vi "WhileLoop to Code.vi"(8 "error in":errorcluster, 10 "C code in":string, 11 "WhileLoop ref":refnum<vi>) -> (0 "error out":errorcluster, 2 "C code":string, 3 "terminals info":T1)   [LabVIEW 2014]
uses:
  <vilib>/regexp/Match Regular Expression.xnode
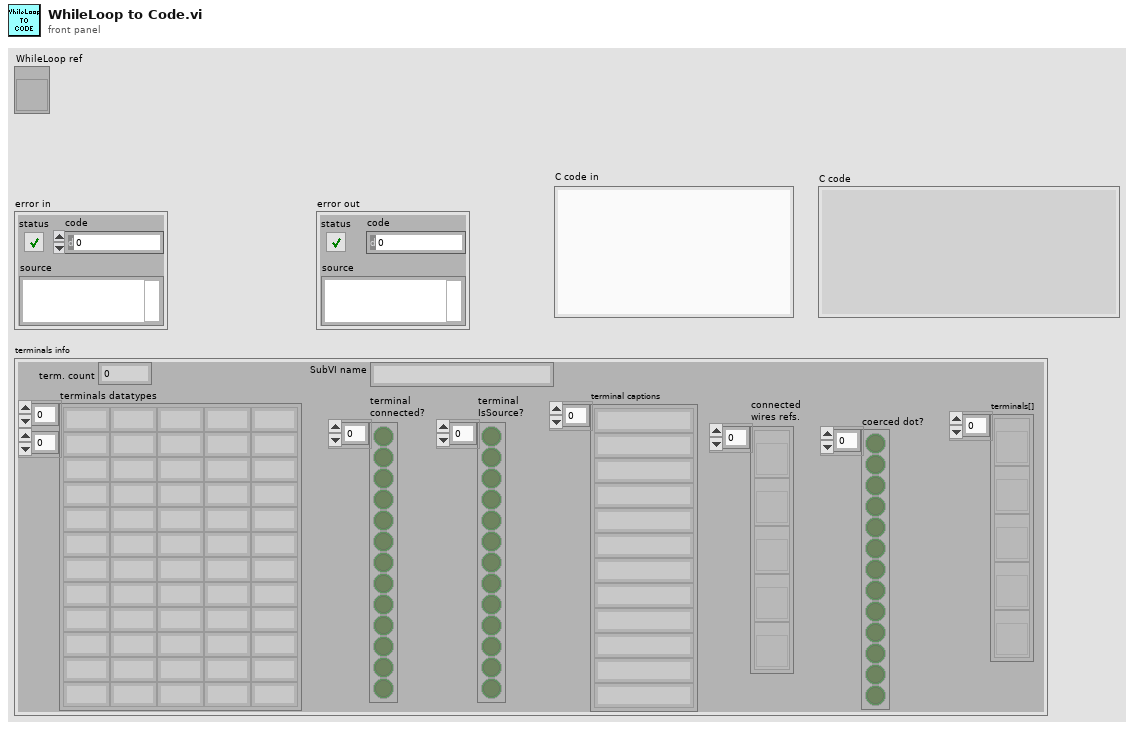
[diagram p1: front panel]
types:
  T1 = cluster{"terminals datatypes":string[][], "terminal\nconnected?":bool[], "terminal captions":string[], "term. count":i32, "terminal\nIsSource?":bool[], "SubVI name":string, "connected\nwires refs.":refnum<vi>[], "coerced dot?":bool[], "terminals[]":refnum<vi>[]}
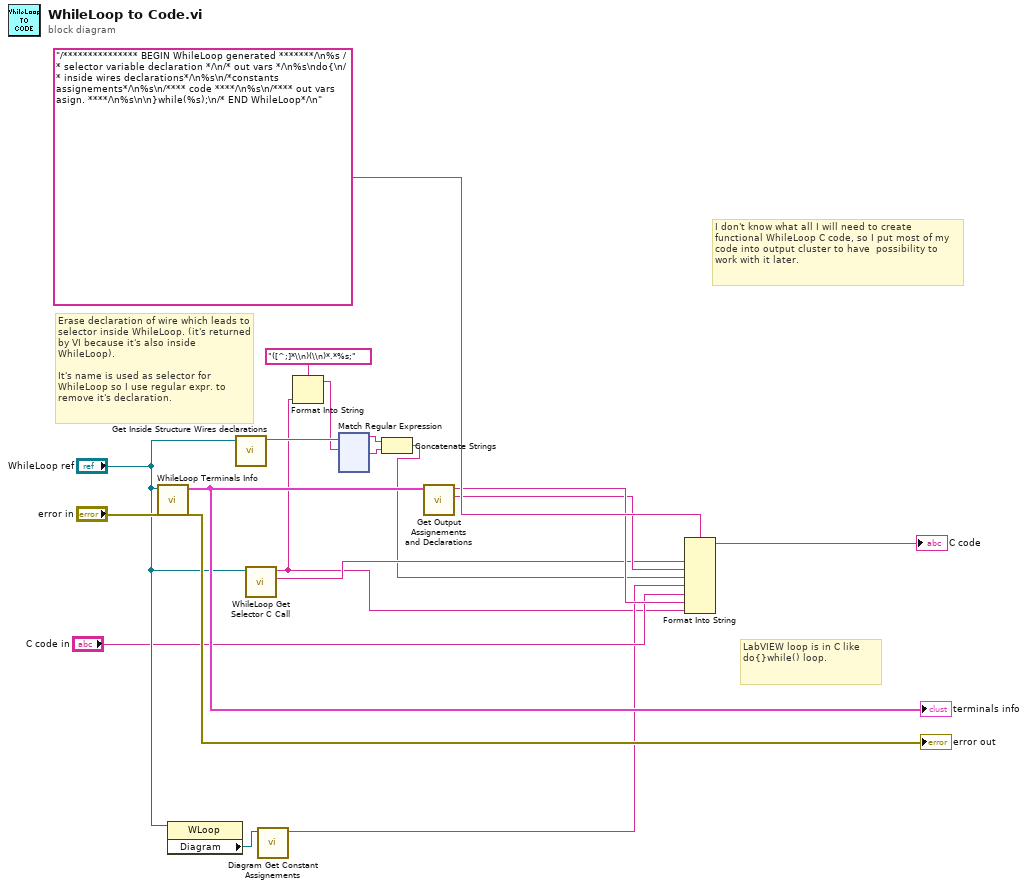
[diagram p0: block diagram]
diagram:
  # "Erase declaration of wire which leads to selector inside WhileLoop. (it's returned by VI because it's also inside WhileLoop).\n\nIt's name is used as selector for WhileLoop so I use regular expr. to remove it's declaration."
  # "I don't know what all I will need to create functional WhileLoop C code, so I put most of my code into output cluster to have  possibility to work with it later."
  # "LabVIEW loop is in C like do{}while() loop."
  n1 = call "WhileLoop Terminals Info.vi"("error in"="error in", "reference"="WhileLoop ref") -> ("error out"=→"error out":errorcluster, "output cluster"=w16:T1)  [unwired: 7 in, 1 out]
  "terminals info" <- w16
  n2 = property on="Property Node" class="WLoop"(reference="WhileLoop ref") -> ("Diagram"=w12:refnum<vi>)  [unwired: 1 in, 2 out]
  n3 = call "Get Inside Structure Wires declarations.vi"("GObject in"="WhileLoop ref") -> ("structure inside wires C declarations"=w7:string)  [unwired: 10 in]
  n4 = call "WhileLoop Get Selector C Call.vi"("reference"="WhileLoop ref") -> ("WhileLoop Selector C declaration"=w8:string, "WhileLoop Selector C var name"=w2:string)  [unwired: 8 in, 1 out]
  n5 = call "Diagram Get Constant Assignements.vi"("Diagram ref."=w12) -> ("Constant assignements to wires"=w9:string)  [unwired: 10 in]
  n6 = Format Into String(format string="([^;]*\\n)(\\n)*.*%s;" ("input string"), w2) -> (resulting string=w3:string)  [unwired: 2 in, 1 out]
  n7 = xnode "Match Regular Expression"("input string"=w7, "regular expression"=w3) -> ("before match"=w6:string, "after match"=w5:string)  [unwired: 4 in, 3 out]
  n8 = Concatenate Strings(w6, w5) -> (w4:string)
  n9 = call "Get Output Assignements and Declarations.vi"("output cluster"=w16) -> ("output declarations"=w14:string, "outuput assignements"=w15:string)  [unwired: 8 in, 1 out]
  n10 = Format Into String(format string="/*************** BEGIN WhileLoop generated *******/\n%s /* selector variable declaration */\n/* out vars */\n%s\ndo{\n/* inside wires declarations*/\n%s\n/*constants assignements*/\n%s\n/**** code ****/\n%s\n/**** out vars asign. ****/\n%s\n\n}while(%s);\n/* END WhileLoop*/\n", w8, w14, w4, w9, "C code in", w15, w2) -> (resulting string=→"C code":string)  [unwired: 2 in, 1 out]
